vi "Erase Curve.vi"(7 "Erase Curve (T: Yes)":bool=TRUE, 8 "error in (no error)":errorcluster, 10 "Curve to Erase (21)":dbl=21.0, 11 "VISA resource name":refnum<visa-resource-name>) -> (0 "error out":errorcluster, 3 "VISA resource name out":refnum<visa-resource-name>)   [LabVIEW 2020, in "Lake Shore 336.lvlib"]
doc: "This VI erases a user curve. Erasing the curve sets all identification parameters to default and blanks all breakpoint values."
uses:
  Lake Shore 336.lvlib
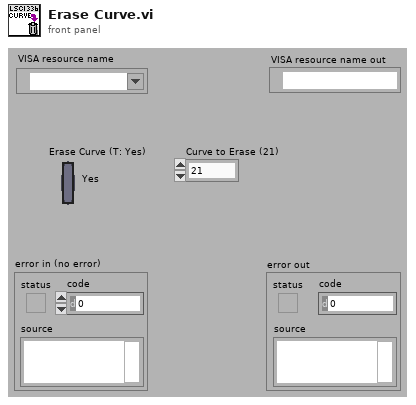
[diagram p1: front panel]
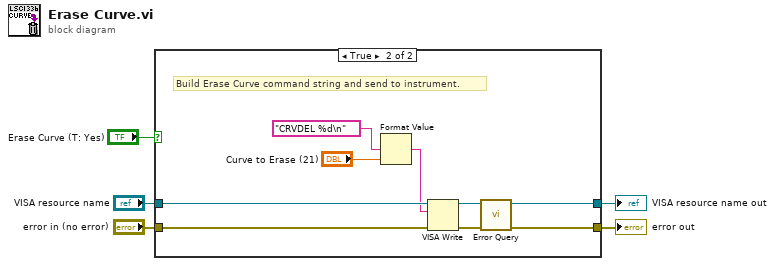
[diagram p0: block diagram]
diagram:
  n1 = case shown="True" "Erase Curve (T: Yes)" {
    tunnel: "VISA resource name" -> [w7 w16]
    tunnel: "error in (no error)" -> [w6 w15]
    tunnel: [w7 w12] -> w3
    tunnel: [w6 w11] -> w2
    frame False {
      # "Do not erase curve"
    }
    frame True {
      # "Build Erase Curve command string and send to instrument."
      n2 = Format Value(format string="CRVDEL %d\n", value (0)="Curve to Erase (21)") -> (output string=w9:string)  [unwired: 1 in]
      n3 = VISA Write(VISA resource name=w16, write buffer=w9, error in (no error)=w15) -> (VISA resource name out=w13:refnum<visa-resource-name>, error out=w14:errorcluster)  [unwired: 1 out]
      n4 = call "Error Query.vi"("error in (no error)"=w14, "VISA resource name"=w13) -> ("error out"=w11:errorcluster, "VISA resource name out"=w12:refnum<visa-resource-name>)  [unwired: 7 in, 1 out]
    }
  }
  "VISA resource name out" <- w3
  "error out" <- w2
